vi "Model Calibration Control - 2D Table.vi"() -> ()   [LabVIEW 2011]
doc: "Sample numeric display item."
uses:
  <vilib>/NI Veristand/Display Template Support/Display Template Support.llb/cluster_Screen Item Settings.ctl
  <vilib>/NI Veristand/Display Template Support/Display Template Support.llb/cluster_Graph Scale Settings.ctl
  <vilib>/NI Veristand/Display Template Support/Display Template Support.llb/cluster_Graph Plot Settings.ctl
  Tables/TBL2D.xctl
  NationalInstruments.VeriStand.SystemStorage
  <vilib>/NI Veristand/Display Template Support/Display Template Support.llb/enum_Display Template Handler Minimal To Widget Msg.ctl
  <vilib>/NI Veristand/Display Template Support/Display Template Support.llb/enum_Display Template Handler Minimal To Workspace.ctl
  Tables/Limits TBL2D.ctl
  <vilib>/NI Veristand/Execution/Workspace/SystemState.ctl
  <vilib>/NI Veristand/Display Template Support/Display Template Support.llb/sub_Display Template Handler Custom.vi
  <vilib>/NI Veristand/Execution/ModelManager/NI VeriStand - Set Parameter 2D Array Values.vi
  <vilib>/NI Veristand/Execution/Workspace/NI VeriStand - Get Multiple Channel Values.vi
  <vilib>/NI Veristand/Execution/Workspace/NI VeriStand - Get Single Channel Value.vi
  <vilib>/NI Veristand/Execution/ModelManager/NI_VS ModelManager ExecutionAPI.lvlib
  <vilib>/NI Veristand/Execution/Workspace/NI_VS Workspace ExecutionAPI.lvlib
panel:
  in  "Paths":string[](array[string])
  out "Selected Parameter":string
  in  "NIVS.System Definition Root":refnum<k24>
  in  "TBL2D":cluster{"X":sgl[], "Y":sgl[], "Z":sgl[][]}(xcontrol)
  in  "Item.Data":T1
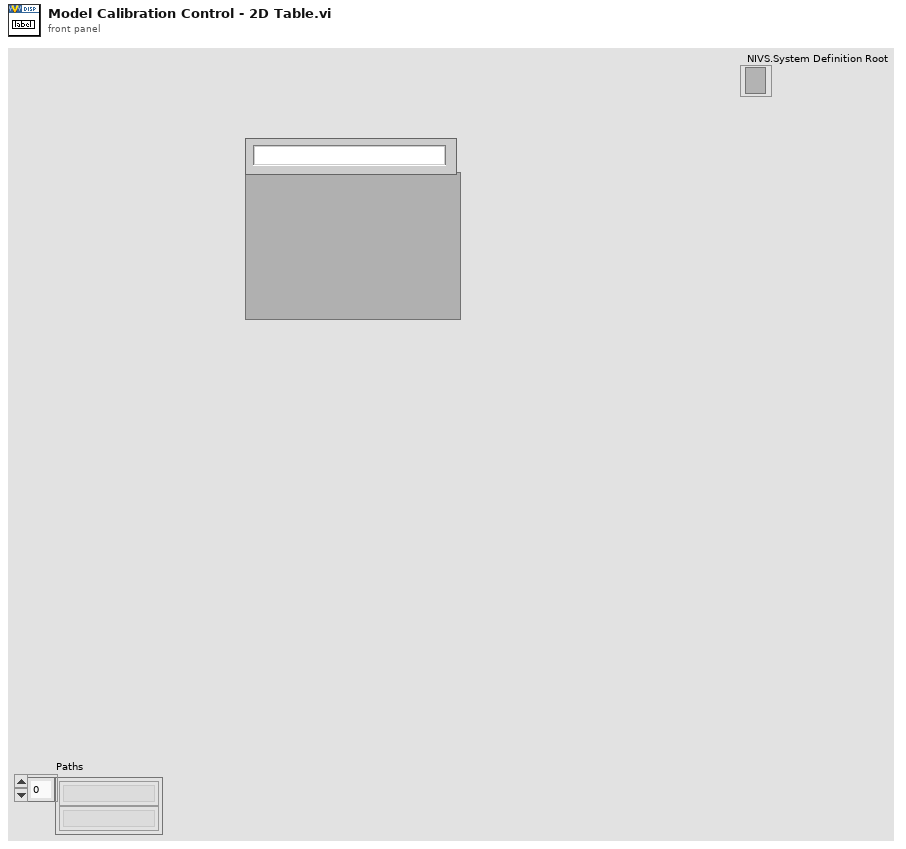
[diagram p1: front panel]
types:
  T1 = typedef "cluster_Screen Item Settings.ctl" = cluster{"Template VI":string, "Position X":i32, "Position Y":i32, "Custom":string, "Show Title Bar":bool, "ID":i32, "Always On Top":bool, "Allow Resize":bool, "Allow Minimize":bool, "Allow Close":bool, "Size to Screen":bool, "Screen.ID":i32, "State":enum16{"Normal", "New"}, "Title":string, "Window Bounds":cluster{"[0]":i16, "[1]":i16, "[2]":i16, "[3]":i16}, "Channel Ref":u64, "Unit":string, "Default Units?":bool, "Flash Limit?":bool, "Color 1":u32, "Color 2":u32, "Color 3":u32, "Color 4":u32, "Bck Color":u32, "Fore Color":u32, "Limit 1":dbl, "Limit 2":dbl, "Limit 3":dbl, "Limit 4":dbl, "Limit Mode 1":i32, "Limit Mode 2":i32, "Limit Mode 3":i32, "Limit Mode 4":i32, "Scale Precision":i32, "Scale Min":dbl, "Scale Max":dbl, "Format":i32, "Precision":i32, "Background Type":i32, "IDs":i32[], "Units":string[], "Labels":string[], "Scale Factor":dbl, "Scale Offset":dbl, "YScale Index":u32[], "XScale":T2, "YScales":T2[], "Plots":T3[], "Update Period":dbl, "History Length":dbl, "My.Ref":refnum<vi>, "Is Control?":bool, "Channel Paths":string[], "Custom Data":variant}
  T2 = typedef "cluster_Graph Scale Settings.ctl" = cluster{"Format":u8, "Precision":u8, "Fit":u8, "Label":string, "Use Default Label":bool, "Label Visible":bool, "Min":dbl, "Max":dbl}
  T3 = typedef "cluster_Graph Plot Settings.ctl" = cluster{"Bar Style":u8, "Fill To":i16, "Fill/PtColor":u32, "Line Style":u8, "Line Width":u8, "Color":u32, "Interp":u8, "Point Style":u8}
  T4 = typedef "TBL2D.xctl/Limits TBL2D.ctl" = cluster{"Min X":sgl, "Max X":sgl, "MaxDiff X":sgl, "MaxGrad X":sgl, "Min Y":sgl, "Max Y":sgl, "MaxDiff Y":sgl, "MaxGrad Y":sgl, "Min Z":sgl, "Max Z":sgl, "MaxDiff Z":sgl}
  T5 = typedef "enum_Display Template Handler Minimal To Workspace.ctl" = cluster{"Operation":enum16{"SetCustomData", "DeleteItem"}, "Data":variant}
  T6 = typedef "enum_Display Template Handler Minimal To Widget Msg.ctl" = enum16{"Stop", "LaunchConfigDialog"}
  T7 = typedef "NI_VS ModelManager ExecutionAPI.lvlib/ModelManagerAPI.ctl" = refnum<k24>
  T8 = typedef "NI_VS Workspace ExecutionAPI.lvlib/WorkspaceAPI.ctl" = refnum<k24>
  T9 = typedef "NI_VS Workspace ExecutionAPI.lvlib/SystemState.ctl" = u8
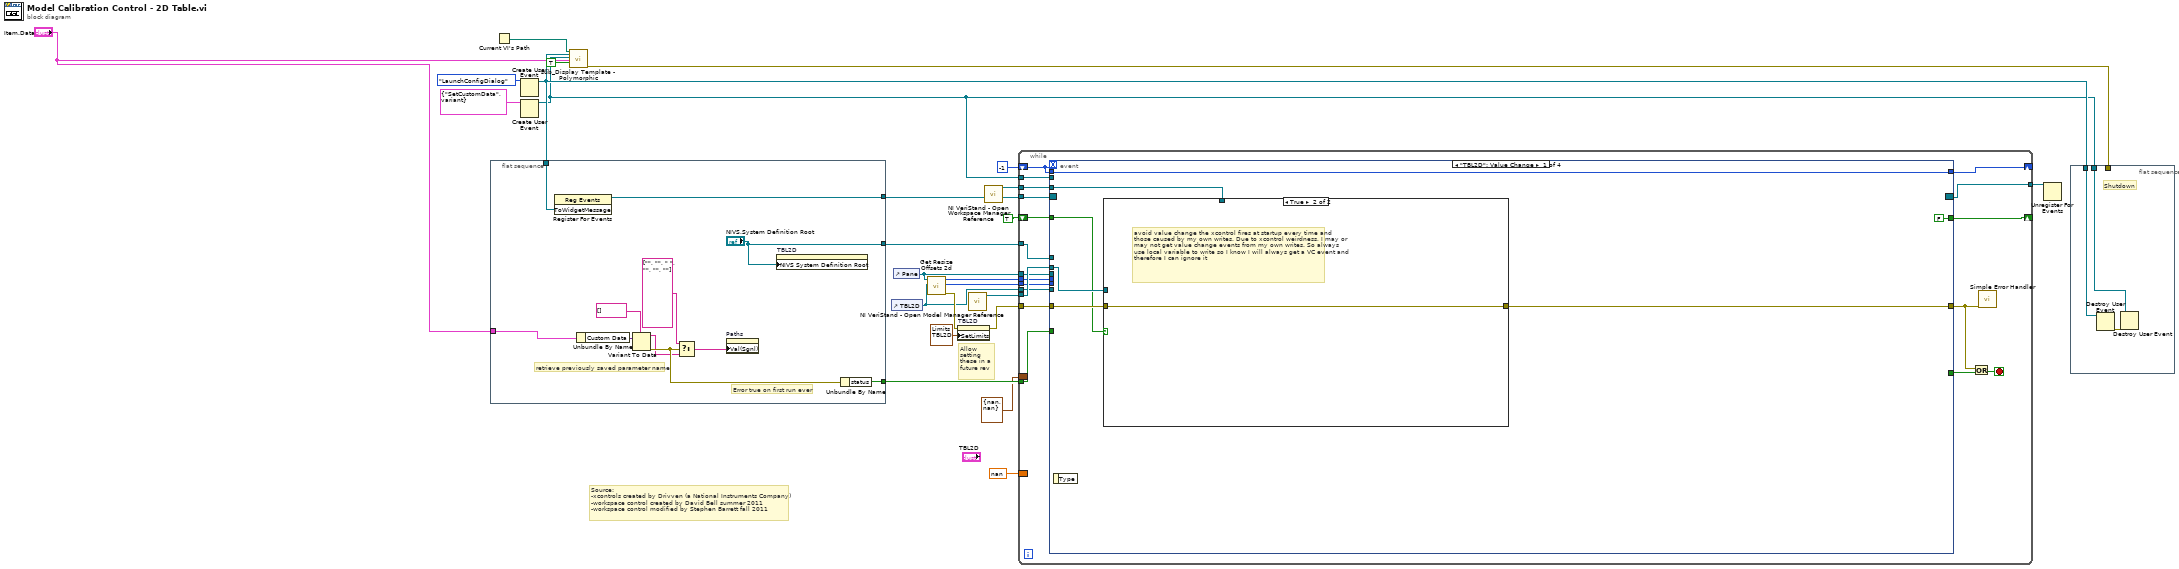
[diagram p0: block diagram]
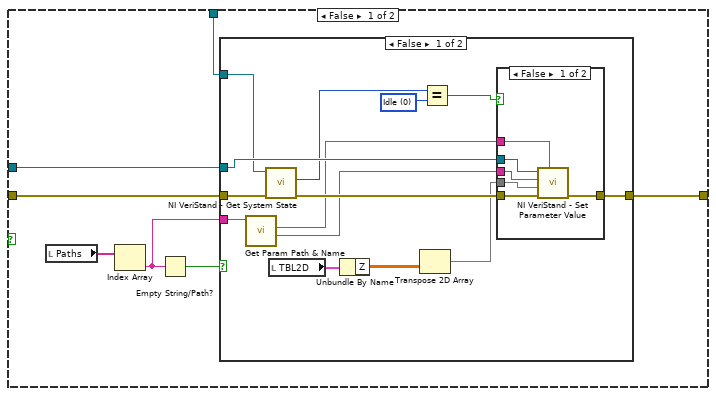
[diagram p2: hidden frame]
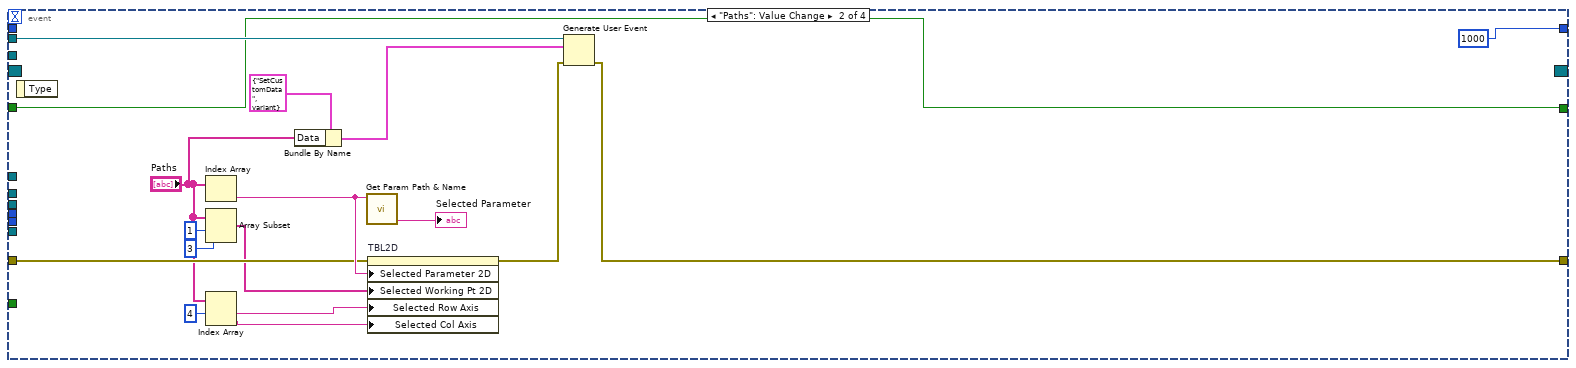
[diagram p5: hidden frame]
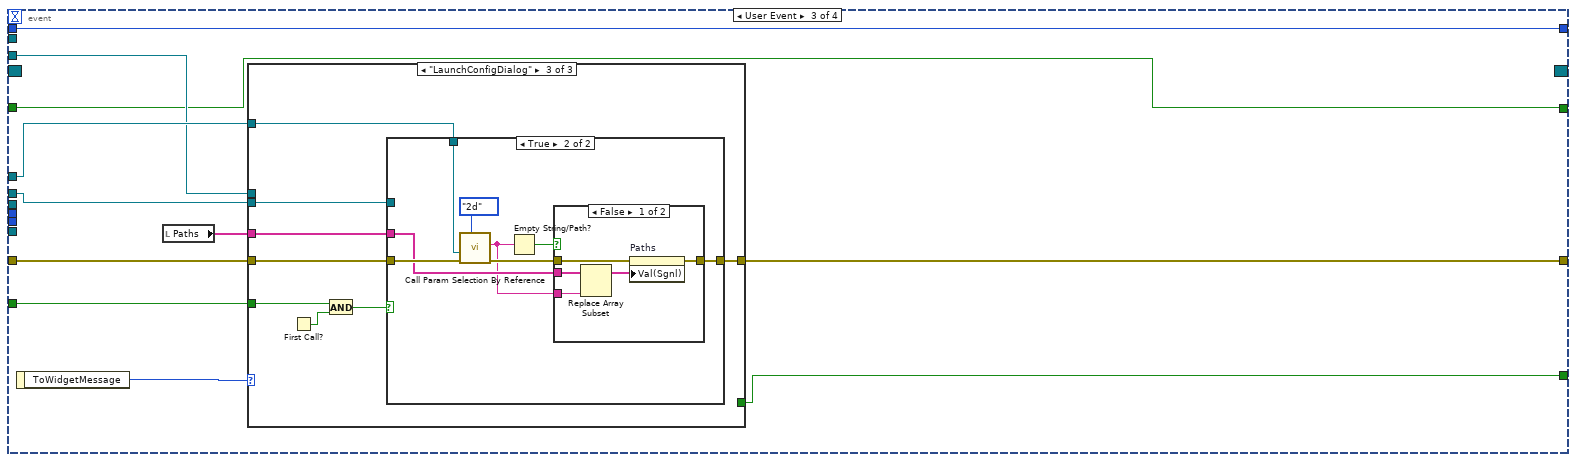
[diagram p6: hidden frame]
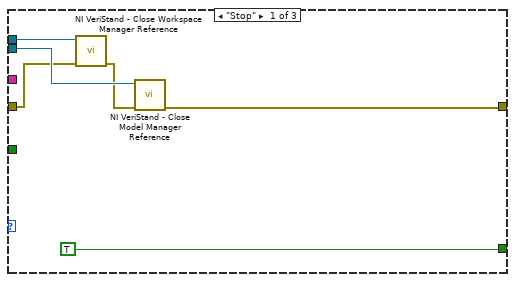
[diagram p7: hidden frame]
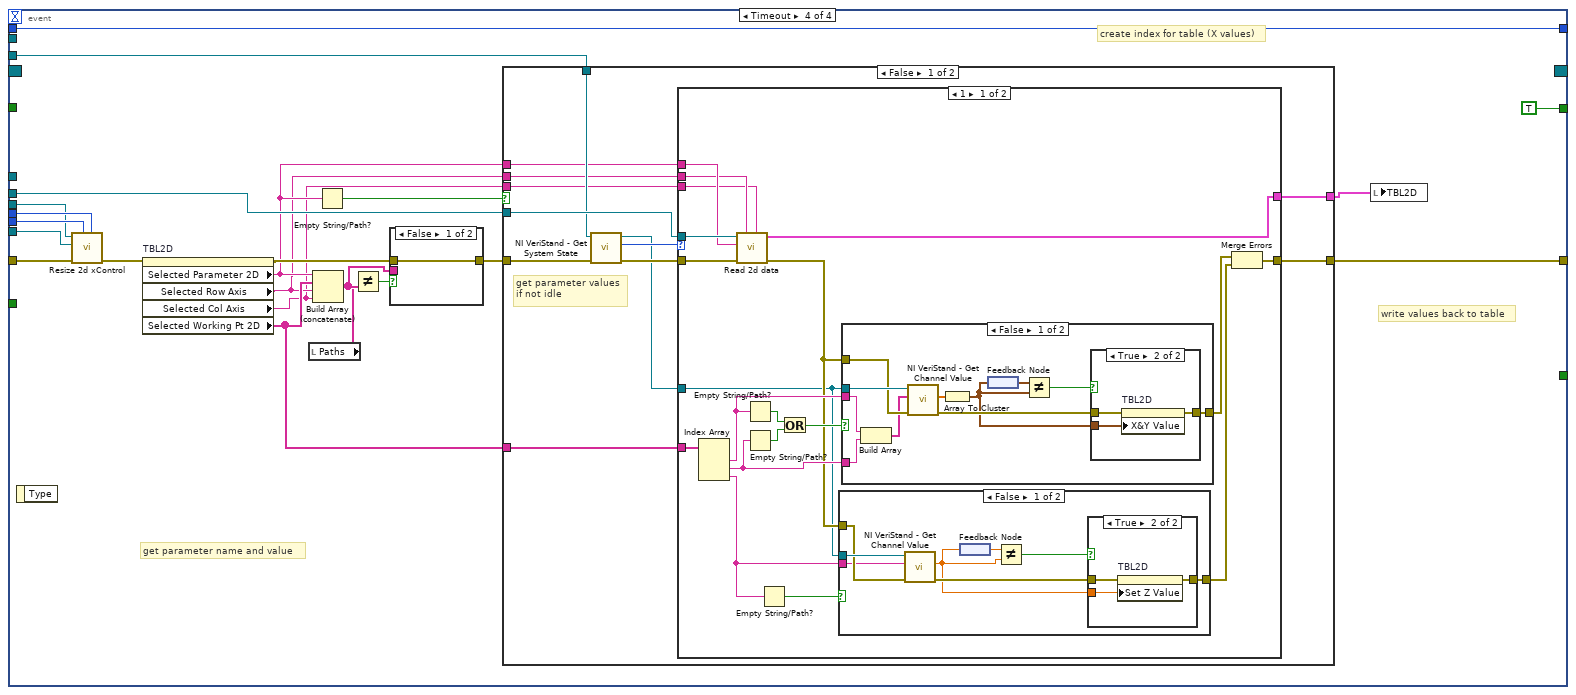
[diagram p11: hidden frame]
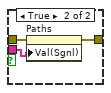
[diagram p12: hidden frame]
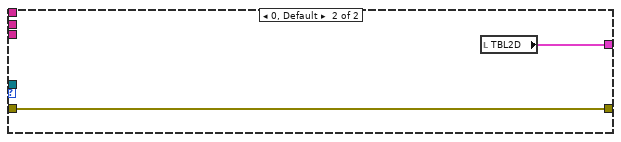
[diagram p17: hidden frame]
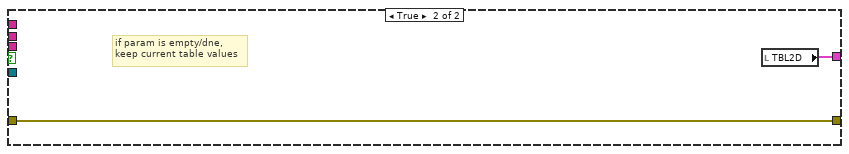
[diagram p18: hidden frame]
diagram:
  # "Source: \n-xcontrols created by Drivven (a National Instruments Company)\n-workspace control created by David Bell summer 2011\n-workspace control modified by Stephen Barrett fall 2011"
  # "Allow setting these in a future rev"
  n1 = flat-sequence {
    tunnel: [w36] -> w23
    tunnel: w22 -> [w35]
    tunnel: "Item.Data" -> [w33]
    tunnel: ["NIVS.System Definition Root"] -> w13
    tunnel: [w28] -> w12
    frame #0 {
      # "Error true on first run ever"
      # "retrieve previously saved parameter name"
      n2 = register-events(w35) -> (reference out=w36:refnum<event-registration>)  [unwired: 2 in, 1 out]
      n3 = Unbundle By Name(w33) -> ("Custom Data"=w34:variant)
      n4 = Variant To Data(type=string[] [], Variant=w34) -> (data=w26:string[], error out=w29:errorcluster)  [unwired: 1 in]
      n5 = Select(t=string[] ["", "", " ", "", "", ""], s=w29, f=w26) -> (s? t:f=w27:string[])
      n6 = property on="Paths" class="Arr (strict)"("Val(Sgnl)"=w27) -> ()  [unwired: 2 in, 2 out]
      n7 = property on="TBL2D" class="TBL2D (strict)"("NIVS System Definition Root"="NIVS.System Definition Root") -> ()  [unwired: 2 in, 2 out]
      n8 = Unbundle By Name(w29) -> ("status"=w28:bool)
    }
  }
  n9 = Current VI's Path() -> (path=w20:path)
  n10 = Create User Event(user event datatype=enum_Display_Template_Handler_Minimal_To_Widget_Msg."LaunchConfigDialog" ("ToWidgetMessage")) -> (user event=w22:refnum<user-event>)  [unwired: 1 in, 1 out]
  n11 = Create User Event(user event datatype=T5 {"Operation"=enum."SetCustomData", "Data"=variant} ("Data")) -> (user event=w19:refnum<user-event>)  [unwired: 1 in, 1 out]
  n12 = call-poly <vilib>:"sub_Display Template - Polymorphic.vi"("Parent.Path"=w20, "ToWidgetEvent"=w22, "ToWorkspace"=w19, "Item.Data"="Item.Data", "Resizable"=TRUE) -> ("error out"=w25:errorcluster)  [unwired: 1 in, 13 out]
  n13 = control-ref of="TBL2D"() -> (w4:refnum<vi>)
  n14 = control-ref of="Pane"() -> (w5:refnum<vi>)
  n15 = call "Get Resize Offsets 2d.vi"("TBL2D Refnum"=w4, "Pane in"=w5) -> ("error out"=w8:errorcluster, "Width Offset"=w7:u32, "Height Offset"=w6:u32)  [unwired: 7 in]
  n16 = property on="TBL2D" class="TBL2D (strict)"(error in=w8, "SetLimits"=T4 {"Min X"=-inf, "Max X"=inf, "MaxDiff X"=inf, "MaxGrad X"=inf, "Min Y"=-inf, "Max Y"=inf, "MaxDiff Y"=inf, "MaxGrad Y"=inf, "Min Z"=-inf, "Max Z"=inf, "MaxDiff Z"=inf}) -> (error out=w11:errorcluster)  [unwired: 1 in, 1 out]
  n17 = call <vilib>:"NI VeriStand - Open Model Manager Reference.vi"() -> ("ModelManager"=w17:T7)  [unwired: 10 in, 1 out]
  n18 = call <vilib>:"NI VeriStand - Open Workspace Manager Reference.vi"() -> ("WorkspaceManager"=w16:T8)  [unwired: 10 in, 1 out]
  n19 = while {
    tunnel: w23 -> [w55]
    tunnel: [w54] -> w14
    tunnel: w19 -> [w51]
    tunnel: w17 -> [w53]
    tunnel: w11 -> [w52]
    tunnel: w16 -> [w50]
    tunnel: w13 -> [w49]
    tunnel: w12 -> [w48]
    border: cluster{"X":sgl, "Y":sgl} {"X"=nan, "Y"=nan} ("X&Y Value") -> [_]
    tunnel: w7 -> [w44]
    tunnel: w6 -> [w43]
    tunnel: w5 -> [w42]
    tunnel: w4 -> [w41]
    border: sgl nan ("Y") -> [_]
    shift-right: [w39] -> _
    shift-left: -1 -> [w40]
    shift-right: [w38] -> _
    shift-left: TRUE -> [w37]
    stop <- w46 stop-if-true
    n20 = event shown="[0] \"TBL2D\": Value Change" {
      selector: w55 -> [_ _ _ _]
      dyn-events: [_ _ _ _] -> w54
      timeout: w40 -> [_ _ _ _]
      tunnel: w53 -> [w61 _ w114 w172]
      tunnel: w52 -> [w62 w104 w119 w163]
      tunnel: w51 -> [_ w105 _ _]
      tunnel: [w59 w103 w112 w154] -> w45
      tunnel: w50 -> [w60 _ w115 w171]
      tunnel: [_ _ w113 _] -> w47
      tunnel: w49 -> [_ _ w116 _]
      tunnel: w48 -> [_ _ w118 _]
      tunnel: w44 -> [_ _ _ w161]
      tunnel: w43 -> [_ _ _ w160]
      tunnel: w42 -> [_ _ _ w159]
      tunnel: w41 -> [_ _ _ w158]
      tunnel: w40 -> [w58 _ w111 w153]
      tunnel: [w58 1000 w111 w153] -> w39
      tunnel: [FALSE w93 w110 TRUE] -> w38
      tunnel: w37 -> [w57 w93 w110 _]
      event "TBL2D": Value Change {
        n21 = event-data() -> ()  [unwired: 1 in, 1 out]
        n22 = case shown="True" w57 {
          tunnel: w62 -> [w69 w92]
          tunnel: w61 -> [w68 _]
          tunnel: w60 -> [w67 _]
          tunnel: [w66 w92] -> w59
          frame False {
            n23 = local read "Paths"() -> (w65:string[])
            n24 = Index Array(array=w65) -> (element=w64:string)  [unwired: 1 in]
            n25 = Empty String/Path?(string/path=w64) -> (empty?=w63:bool)
            n26 = case shown="False" w63 {
              tunnel: [w82 w91] -> w66
              tunnel: w69 -> [w78 w91]
              tunnel: w68 -> [w83 _]
              tunnel: w67 -> [w81 _]
              tunnel: w64 -> [w79 _]
              frame False {
                w76 = T9 0 items=["Idle", "Active"] ("System State")
                n27 = call "Get Param Path & Name.vi"("Path"=w79) -> ("Parameter Path"=w72:string, "Controller name"=w71:string)  [unwired: 8 in, 1 out]
                n28 = call <vilib>:"NI VeriStand - Get System State.vi"("error in (no error)"=w78, "WorkspaceManager in"=w81) -> ("error out"=w77:errorcluster, "System State"=w80:T9)  [unwired: 5 in, 3 out]
                n29 = local read "TBL2D"() -> (w75:cluster{"X":sgl[], "Y":sgl[], "Z":sgl[][]})
                n30 = Unbundle By Name(w75) -> ("Z"=w74:sgl[][])
                n31 = Transpose 2D Array(2D array=w74) -> (transposed array=w73:sgl[][])
                n32 = Equal?(x=w80, y=w76) -> (x = y?=w70:bool)
                n33 = case shown="False" w70 {
                  tunnel: w83 -> [w89 _]
                  tunnel: [w88 w90] -> w82
                  tunnel: w72 -> [w87 _]
                  tunnel: w73 -> [w86 _]
                  tunnel: w77 -> [w85 w90]
                  tunnel: w71 -> [w84 _]
                  frame False {
                    n34 = call-poly <vilib>:"NI VeriStand - Set Parameter Value.vi"("Target"=w84, "error in (no error)"=w85, "Values"=w86, "Parameter"=w87, "ModelManager in"=w89) -> ("error out"=w88:errorcluster)  [unwired: 5 in, 1 out]
                  }
                  frame True {
                  }
                }
              }
              frame True {
              }
            }
          }
          frame True {
            # "avoid value change the xcontrol fires at startup every time and those caused by my own writes. Due to xcontrol weirdness, I may or may not get value change events from my own writes. So always use local variable to write so I know I will always get a VC event and therefore I can ignore it"
          }
        }
      }
      event "Paths": Value Change {
        n35 = event-data() -> ()  [unwired: 1 in, 1 out]
        n36 = Index Array(array="Paths") -> (element=w109:string)  [unwired: 1 in]
        n37 = Array Subset(array="Paths", index=1, length=3) -> (w100:string[])
        n38 = Index Array(array="Paths", index #1=4 ("index")) -> (element #1=w96:string, element #2=w95:string)  [unwired: 1 in]
        n39 = Bundle By Name(cluster=T5 {"Operation"=enum."SetCustomData", "Data"=variant} ("event data"), "Data"="Paths") -> (w106:T5)
        n40 = call "Get Param Path & Name.vi"("Path"=w109) -> ("Last Part"=→"Selected Parameter":string)  [unwired: 8 in, 2 out]
        n41 = property on="TBL2D" class="TBL2D (strict)"(error in=w104, "Selected Parameter 2D"=w109, "Selected Working Pt 2D"=w100, "Selected Row Axis"=w96, "Selected Col Axis"=w95) -> (error out=w108:errorcluster)  [unwired: 1 in, 1 out]
        n42 = Generate User Event(user event=w105, event data cluster=w106, error in=w108) -> (error out=w103:errorcluster)  [unwired: 1 out]
      }
      event User Event {
        n43 = event-data() -> ("ToWidgetMessage"=w120:T6)  [unwired: 1 in]
        n44 = local read "Paths"() -> (w117:string[])
        n45 = case shown="\"LaunchConfigDialog\"" w120 {
          tunnel: [TRUE ("1-D array?") _ _] -> w113
          tunnel: w114 -> [w124 _ w135]
          tunnel: w116 -> [_ _ w134]
          tunnel: w115 -> [w125 _ _]
          tunnel: w117 -> [_ _ w131]
          tunnel: w119 -> [w123 w127 w133]
          tunnel: [w121 w127 w132] -> w112
          tunnel: w118 -> [_ _ w130]
          frame "Stop" {
            n46 = call <vilib>:"NI VeriStand - Close Workspace Manager Reference.vi"("error in (no error)"=w123, "WorkspaceManager"=w125) -> ("error out"=w122:errorcluster)  [unwired: 9 in]
            n47 = call <vilib>:"NI VeriStand - Close Model Manager Reference.vi"("error in (no error)"=w122, "ModelManager"=w124) -> ("error out"=w121:errorcluster)  [unwired: 9 in]
          }
          frame Default {
          }
          frame "LaunchConfigDialog" {
            n48 = First Call?() -> (First Call?: T/F=w128:bool)
            n49 = And(x=w130, y=w128) -> (x .and. y?=w129:bool)
            n50 = case shown="True" w129 {
              tunnel: w135 -> [_ _]
              tunnel: w134 -> [_ w144]
              tunnel: w131 -> [_ w139]
              tunnel: w133 -> [w136 w143]
              tunnel: [w136 w140] -> w132
              frame False {
              }
              frame True {
                n51 = call "Call Param Selection By Reference.vi"("Param Size"=enum16{"Scalar", "1d", "2d"}."2d", "error in (no error)"=w143, "NIVS.System Definition Root"=w144) -> ("error out"=w141:errorcluster, "Selected NodePath"=w138:string)  [unwired: 7 in]
                n52 = Empty String/Path?(string/path=w138) -> (empty?=w137:bool)
                n53 = case shown="False" w137 {
                  tunnel: w141 -> [w149 w150]
                  tunnel: [w147 w150] -> w140
                  tunnel: w139 -> [w146 _]
                  tunnel: w138 -> [w145 _]
                  frame False {
                    n54 = Replace Array Subset(array=w146, new element=w145) -> (w148:string[])  [unwired: 1 in]
                    n55 = property on="Paths" class="Arr (strict)"(error in=w149, "Val(Sgnl)"=w148) -> (error out=w147:errorcluster)  [unwired: 1 in, 1 out]
                  }
                  frame True {
                  }
                }
              }
            }
          }
        }
      }
      event Timeout {
        # "write values back to table"
        # "create index for table (X values)"
        # "get parameter name and value"
        n56 = event-data() -> ()  [unwired: 1 in, 1 out]
        n57 = call "Resize 2d xControl.vi"("Height Offset"=w160, "Width Offset"=w161, "error in (no error)"=w163, "Control in"=w158, "Pane"=w159) -> ("error out"=w162:errorcluster)  [unwired: 6 in]
        n58 = property on="TBL2D" class="TBL2D (strict)"(error in=w162) -> (error out=w167:errorcluster, "Selected Parameter 2D"=w164:string, "Selected Row Axis"=w156:string, "Selected Col Axis"=w155:string, "Selected Working Pt 2D"=w157:string[])  [unwired: 1 in, 1 out]
        n59 = local read "Paths"() -> (w166:string[])
        n60 = Build Array (concatenate)(w164, w157, w156, w155) -> (w169:string[])
        n61 = Empty String/Path?(string/path=w164) -> (empty?=w170:bool)
        n62 = Not Equal?(x=w169, y=w166) -> (x != y?=w168:bool)
        n63 = case shown="False" w168 {
          tunnel: w167 -> [w173 w176]
          tunnel: [w173 w175] -> w165
          tunnel: w169 -> [_ w174]
          frame False {
          }
          frame True {
            n64 = property on="Paths" class="Arr (strict)"(error in=w176, "Val(Sgnl)"=w174) -> (error out=w175:errorcluster)  [unwired: 1 in, 1 out]
          }
        }
        n65 = case shown="False" w170 {
          tunnel: [w183 w240] -> w154
          tunnel: [w182 w239] -> w151
          tunnel: w172 -> [w188 _]
          tunnel: w165 -> [w186 w240]
          tunnel: w164 -> [w179 _]
          tunnel: w171 -> [w187 _]
          tunnel: w157 -> [w181 _]
          tunnel: w156 -> [w178 _]
          tunnel: w155 -> [w177 _]
          frame False {
            # "get parameter values\nif not idle"
            n66 = call <vilib>:"NI VeriStand - Get System State.vi"("error in (no error)"=w186, "WorkspaceManager in"=w187) -> ("error out"=w185:errorcluster, "System State"=w184:T9, "WorkspaceManager  out"=w180:T8)  [unwired: 5 in, 2 out]
            n67 = case shown="1" w184 {
              tunnel: w188 -> [w207 _]
              tunnel: [w199 w237] -> w182
              tunnel: w185 -> [w206 w238]
              tunnel: [w195 w238] -> w183
              tunnel: w181 -> [w202 _]
              tunnel: w180 -> [w196 _]
              tunnel: w179 -> [w191 _]
              tunnel: w178 -> [w190 _]
              tunnel: w177 -> [w189 _]
              frame 1 {
                n68 = Index Array(array=w202) -> (element #1=w201:string, element #2=w200:string, element #3=w193:string)  [unwired: 3 in]
                n69 = call "Read 2d data.vi"("Col Param Path"=w189, "Row Param Path"=w190, "error in (no error)"=w206, "Parameter Path"=w191, ".NET Refnum in"=w207) -> ("error out"=w197:errorcluster, "TBL2D"=w199:cluster{"X":sgl[], "Y":sgl[], "Z":sgl[][]})  [unwired: 5 in]
                n70 = Empty String/Path?(string/path=w201) -> (empty?=w204:bool)
                n71 = Empty String/Path?(string/path=w200) -> (empty?=w205:bool)
                n72 = Empty String/Path?(string/path=w193) -> (empty?=w192:bool)
                n73 = Or(x=w204, y=w205) -> (x .or. y?=w203:bool)
                n74 = case shown="False" w192 {
                  tunnel: w196 -> [w215 _]
                  tunnel: w197 -> [w214 w220]
                  tunnel: [w213 w220] -> w194
                  tunnel: w193 -> [w209 _]
                  frame False {
                    n75 = call-poly <vilib>:"NI VeriStand - Get Channel Value.vi"("error in (no error)"=w214, "Channel"=w209, "WorkspaceManager in"=w215) -> ("error out"=w211:errorcluster, "Value"=w210:dbl)  [unwired: 6 in, 1 out]
                    n76 = feedback #1() -> (w212:dbl)
                    n77 = feedback-in #1(w210) -> ()
                    n78 = Not Equal?(x=w212, y=w210) -> (x != y?=w208:bool)
                    n79 = case shown="True" w208 {
                      tunnel: w211 -> [w216 w219]
                      tunnel: [w216 w218] -> w213
                      tunnel: w210 -> [_ w217]
                      frame False {
                      }
                      frame True {
                        n80 = property on="TBL2D" class="TBL2D (strict)"(error in=w219, "Set Z Value"=w217) -> (error out=w218:errorcluster)  [unwired: 1 in, 1 out]
                      }
                    }
                  }
                  frame True {
                  }
                }
                n81 = case shown="False" w203 {
                  tunnel: w201 -> [w226 _]
                  tunnel: w196 -> [w231 _]
                  tunnel: w200 -> [w225 _]
                  tunnel: w197 -> [w230 w236]
                  tunnel: [w229 w236] -> w198
                  frame False {
                    n82 = Build Array(w226, w225) -> (w224:string[])
                    n83 = call-poly <vilib>:"NI VeriStand - Get Channel Value.vi"("error in (no error)"=w230, "Channels"=w224, "WorkspaceManager in"=w231) -> ("error out"=w227:errorcluster, "Values"=w223:dbl[])  [unwired: 6 in, 1 out]
                    n84 = Array To Cluster(array=w223) -> (cluster=w222:cluster{"Values[0]":dbl, "Values[1]":dbl})
                    n85 = feedback #2() -> (w228:cluster{"Values[0]":dbl, "Values[1]":dbl})
                    n86 = feedback-in #2(w222) -> ()
                    n87 = Not Equal?(x=w228, y=w222) -> (x != y?=w221:bool)
                    n88 = case shown="True" w221 {
                      tunnel: w227 -> [w232 w235]
                      tunnel: [w232 w234] -> w229
                      tunnel: w222 -> [_ w233]
                      frame False {
                      }
                      frame True {
                        n89 = property on="TBL2D" class="TBL2D (strict)"(error in=w235, "X&Y Value"=w233) -> (error out=w234:errorcluster)  [unwired: 1 in, 1 out]
                      }
                    }
                  }
                  frame True {
                  }
                }
                n90 = Merge Errors(w198, w194) -> (w195:errorcluster)
              }
              frame 0, Default {
                n91 = local read "TBL2D"() -> (w237:cluster{"X":sgl[], "Y":sgl[], "Z":sgl[][]})
              }
            }
          }
          frame True {
            # "if param is empty/dne,\nkeep current table values"
            n92 = local read "TBL2D"() -> (w239:cluster{"X":sgl[], "Y":sgl[], "Z":sgl[][]})
          }
        }
        n93 = local write "TBL2D"(w151) -> ()
      }
    }
    n94 = Or(x=w45, y=w47) -> (x .or. y?=w46:bool)
    n95 = call <vilib>:"Simple Error Handler.vi"("error in (no error)"=w45) -> ()  [unwired: 4 in, 5 out]
  }
  n96 = Unregister For Events(event registration refnum=w14) -> ()  [unwired: 1 in, 1 out]
  n97 = flat-sequence {
    tunnel: w25 -> [_]
    tunnel: w22 -> [w243]
    tunnel: w19 -> [w241]
    frame #0 {
      # "Shutdown"
      n98 = Destroy User Event(user event=w243) -> (error out=w242:errorcluster)  [unwired: 1 in]
      n99 = Destroy User Event(user event=w241, error in=w242) -> ()  [unwired: 1 out]
    }
  }
